vi "test Sequential Consumer Messages.vi"(8 "error in (no error)":errorcluster, 11 "TestCase in":refnum<class "Multi Consumer Test Case.lvclass">) -> (0 "error out":errorcluster, 3 "TestCase out":refnum<class "Multi Consumer Test Case.lvclass">)   [LabVIEW 2017, in "Multi Consumer Test Case.lvclass"]
uses:
  Multi Consumer Test Case.lvclass
  Support/Messages/Consumer Name Response Message/Consumer Name Response Message.lvclass
  Support/Messages/Consumer Name Request Message/Consumer Name Request Message.lvclass
  C:/github/niveristand-custom-device-message-library/Source/Message/Abstract Message/Abstract Message.lvclass
  Message/Shutdown Message/Shutdown Message.lvclass
  Multi Consumer Test Case.lvclass/Multi Consumer Test Case.ctl
  Support/Messages/Consumer Name Response Message/Consumer Name Response Message.lvclass/Consumer Name Response Message.ctl
  Support/Messages/Consumer Name Response Message/Read Consumer Name.vi
  Producer/Abstract Producer/Abstract Producer.lvclass
  <vilib>/addons/_JKI Toolkits/VI Tester/TestCase.llb/TestCase.lvclass
  C:/Program Files (x86)/National Instruments/LabVIEW 2017/vi.lib/addons/_JKI Toolkits/VI Tester/TestCase.llb/TestCase.lvclass
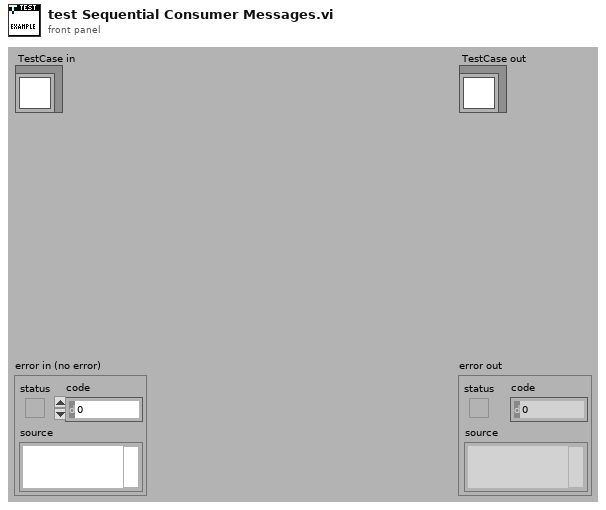
[diagram p1: front panel]
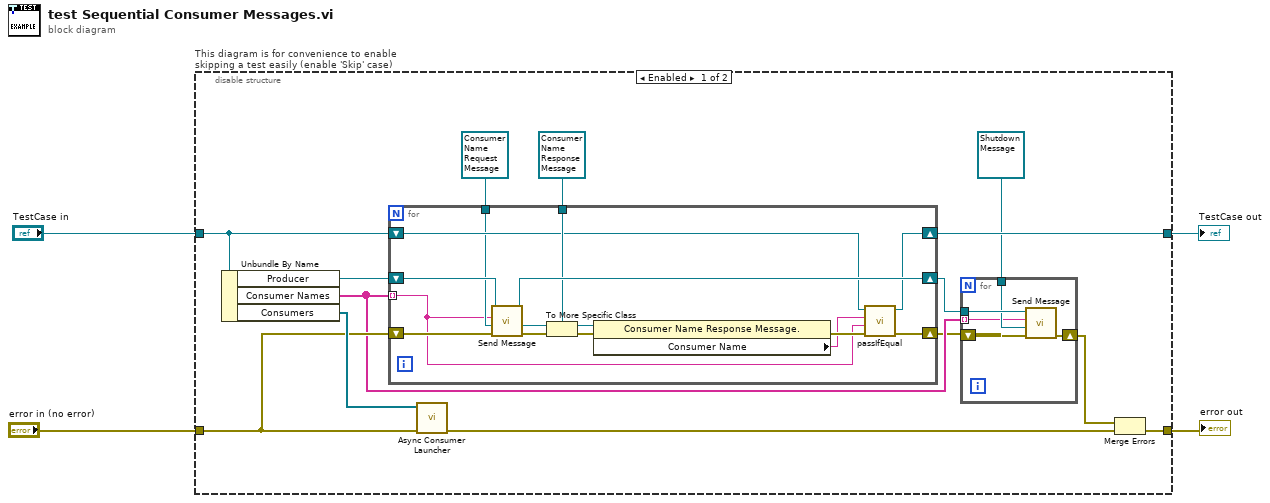
[diagram p0: block diagram]
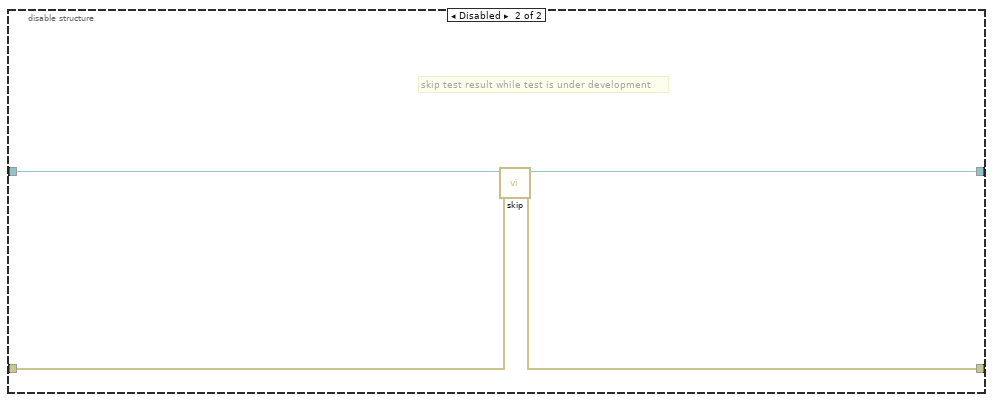
[diagram p2: hidden frame]
diagram:
  n1 = disable-structure "This diagram is for convenience to enable skipping a test easily (enable 'Skip' case)" shown="Enabled" {
    disable-tunnel: "TestCase in" -> [w12 w42]
    disable-tunnel: [w11 w40] -> w1
    disable-tunnel: [w14 w41] -> w3
    disable-tunnel: "error in (no error)" -> [w16 w39]
    frame Enabled {
      n2 = Unbundle By Name(w12) -> ("Producer"=w18:refnum<class "Abstract Producer.lvclass">, "Consumer Names"=w7:string[], "Consumers"=w17:refnum<class "Abstract Consumer.lvclass">[])
      n3 = for {
        tunnel: w7 -> [w24] mode=indexing
        shift-right: [w37] -> w8
        shift-left: w18 -> [w38]
        shift-right: [w29] -> w6
        shift-left: w16 -> [w36]
        tunnel: refnum<class "Consumer Name Response Message.lvclass"> refnum ("Consumer Name Response Message.lvclass") -> [w32]
        shift-right: [w27] -> w11
        shift-left: w12 -> [w28]
        tunnel: refnum<class "Consumer Name Request Message.lvclass"> refnum ("Consumer Name Request Message.lvclass") -> [w25]
        n4 = call-dynamic "Send Message.vi"("error in (no error)"=w36, "Message in"=w25, "Consumer in"=w24, "Abstract Producer in"=w38) -> ("error out"=w35:errorcluster, "Message out"=w33:refnum<class "Abstract Message.lvclass">, "Abstract Producer out"=w37:refnum<class "Abstract Producer.lvclass">)  [unwired: 5 in]
        n5 = To More Specific Class(target class=w32, reference=w33, error in=w35) -> (specific class reference=w31:refnum<class "Consumer Name Response Message.lvclass">, error out=w34:errorcluster)
        n6 = property class="Consumer Name Response Message."(reference=w31, error in=w34) -> (error out=w30:errorcluster, "Consumer Name"=w26:string)  [unwired: 1 out]
        n7 = call-dynamic "passIfEqual.vi"("error in (no error)"=w30, "y"=w24, "x"=w26, "TestCase in"=w28) -> ("error out"=w29:errorcluster, "TestCase out"=w27:refnum<class "Multi Consumer Test Case.lvclass">)  [unwired: 6 in]
      }
      n8 = call "Async Consumer Launcher.vi"("error in (no error)"=w16, "Consumers"=w17) -> ("error out"=w15:errorcluster)  [unwired: 9 in]
      n9 = for {
        shift-right: [w19] -> w5
        shift-left: w6 -> [w22]
        tunnel: w8 -> [w23]
        tunnel: refnum<class "Shutdown Message.lvclass"> refnum ("Messaging.lvlib:Message.lvlib:Shutdown Message.lvclass") -> [w21]
        tunnel: w7 -> [w20] mode=indexing
        n10 = call-dynamic "Send Message.vi"("error in (no error)"=w22, "Message in"=w21, "Consumer in"=w20, "Abstract Producer in"=w23) -> ("error out"=w19:errorcluster)  [unwired: 5 in, 2 out]
      }
      n11 = Merge Errors(w5, w15) -> (w14:errorcluster)
    }
    frame Disabled {
      # "skip test result while test is under development"
      n12 = call <vilib>:"skip.vi"("error in (no error)"=w39, "TestCase in"=w42) -> ("error out"=w41:errorcluster, "TestCase out"=w40:refnum<class "Multi Consumer Test Case.lvclass">)  [unwired: 8 in]
    }
  }
  "error out" <- w3
  "TestCase out" <- w1
